vi "FGV Komm Systemeinstellungen.vi"(0 "Systemeinstellungen":T1, 11 "error in (no error)":errorcluster caption="Fehler (Eingang, kein Fehler)", 13 "Aktion":T2) -> (4 "Systemeinstellungen":T1, 15 "error out":errorcluster caption="Fehler (Ausgang)")   [LabVIEW 2020, in "Allgemein.lvlib"]
uses:
  Allgemein.lvlib
  Cluster Komm Systemeinstellungen.ctl
  Aktion FGV Komm Systemeinstellungen.ctl
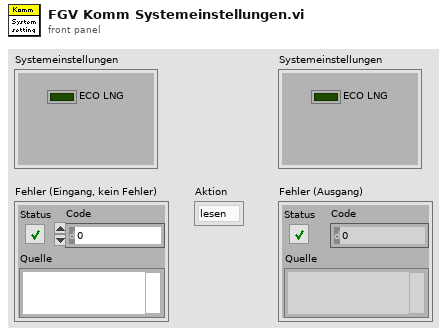
[diagram p1: front panel]
types:
  T1 = typedef "Allgemein.lvlib/Cluster Komm Systemeinstellungen.ctl" = cluster{"ECO LNG":bool}
  T2 = typedef "Allgemein.lvlib/Aktion FGV Komm Systemeinstellungen.ctl" = enum16{"lesen", "schreiben"}
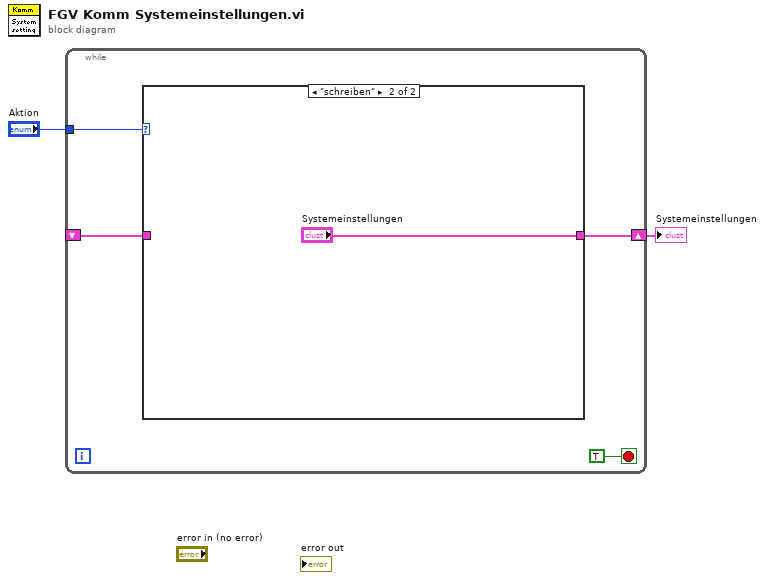
[diagram p0: block diagram]
diagram:
  n1 = while {
    shift-right: [w5] -> w2
    shift-left: _ -> [w4]
    tunnel: "Aktion" -> [w3]
    stop <- TRUE stop-if-true
    n2 = case shown="\"schreiben\"" w3 {
      tunnel: [w7 "Systemeinstellungen"] -> w5
      tunnel: w4 -> [w7 _]
      frame "lesen", Default {
      }
      frame "schreiben" {
      }
    }
  }
  "Systemeinstellungen" <- w2
